vi "GetExpectedCoords.vi"(8 "error in (no error)":errorcluster, 11 "PathTokenizer in":refnum<class "PathTokenizer.lvclass">) -> (0 "error out":errorcluster, 3 "PathTokenizer out":refnum<class "PathTokenizer.lvclass">)   [LabVIEW 2019, in "PathTokenizer.lvclass"]
uses:
  PathTokenizer.lvclass
  PathTokenizer.lvclass/PathTokenizer.ctl
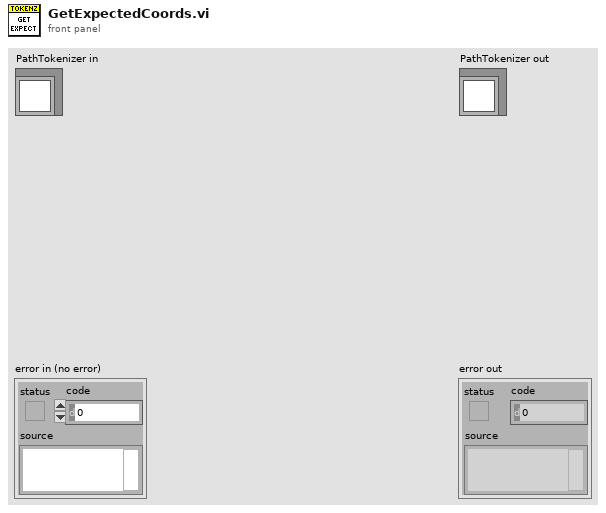
[diagram p1: front panel]
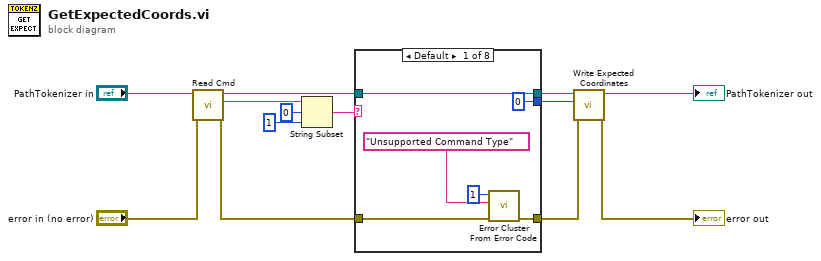
[diagram p0: block diagram]
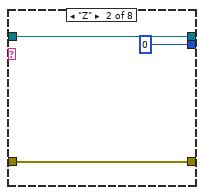
[diagram p2: hidden frame]
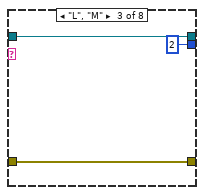
[diagram p3: hidden frame]
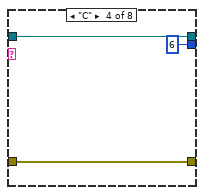
[diagram p4: hidden frame]
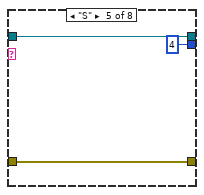
[diagram p5: hidden frame]
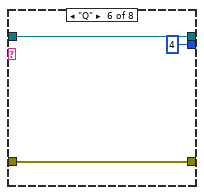
[diagram p6: hidden frame]
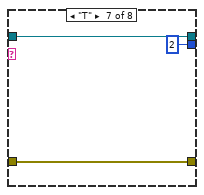
[diagram p7: hidden frame]
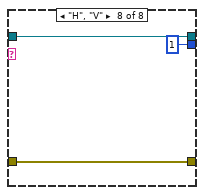
[diagram p8: hidden frame]
diagram:
  n1 = call "Read Cmd.vi"("error in (no error)"="error in (no error)", "PathTokenizer in"="PathTokenizer in") -> ("error out"=w1:errorcluster, "Cmd"=w11:string, "PathTokenizer out"=w8:refnum<class "PathTokenizer.lvclass">)  [unwired: 7 in]
  n2 = String Subset(string=w11, offset (0)=0, length (rest)=1 ("length (rest)")) -> (substring=w6:string)
  n3 = case shown="Default" w6 {
    tunnel: w8 -> [w19 w22 w24 w28 w31 w34 w37 w40]
    tunnel: [w19 w22 w24 w28 w31 w34 w37 w40] -> w7
    tunnel: [w18 w21 w25 w27 w30 w33 w36 w39] -> w4
    tunnel: w1 -> [w17 w21 w25 w27 w30 w33 w36 w39]
    tunnel: [0 0 2 6 4 4 2 1] -> w5
    frame Default {
      n4 = call <vilib>:"Error Cluster From Error Code.vi"("error in (no error)"=w17, "error message (\"\")"="Unsupported Command Type" ("error message (\"\")"), "error code (0)"=1) -> ("error out"=w18:errorcluster)  [unwired: 6 in]
    }
    frame "Z" {
    }
    frame "L", "M" {
    }
    frame "C" {
    }
    frame "S" {
    }
    frame "Q" {
    }
    frame "T" {
    }
    frame "H", "V" {
    }
  }
  n5 = call "Write Expected Coordinates.vi"("error in (no error)"=w4, "Expected Coordinates"=w5, "PathTokenizer in"=w7) -> ("error out"=→"error out":errorcluster, "PathTokenizer out"=→"PathTokenizer out":refnum<class "PathTokenizer.lvclass">)  [unwired: 7 in]
